vi "Aire (subVI).vi"(6 "milliseconds to wait":u32=2000, 8 "error in (no error)":errorcluster, 10 "Gas types":T1(array[ring])=[enum."TVOC", enum."H2S", enum."NO2", enum."O3", enum."SO2", enum."CO", enum."O2", enum."CO2"], 11 "Modbus Master in":refnum<class "Modbus Master.lvclass">) -> (0 "error out":errorcluster, 2 "Measures":dbl[](array[numeric]), 3 "Modbus Master out":refnum<class "Modbus Master.lvclass">)   [LabVIEW 2024]
uses:
  <vilib>/Modbus/master/Modbus Master.lvclass
  C:/Program Files (x86)/National Instruments/LabVIEW 2024/vi.lib/Modbus/subvis/Modbus API/Modbus API.lvclass
  <vilib>/Modbus/subvis/Modbus API/Modbus API.lvclass/Modbus API.ctl
  <vilib>/Modbus/subvis/Transmission Data Unit (ADU)/Transmission Data Unit/Transmission Data Unit.lvclass/Transmission Data Unit.ctl
  <vilib>/Modbus/master/Data Access/Unit ID/Set Unit ID Property.vi
  <vilib>/Modbus/subvis/Transmission Data Unit (ADU)/Transmission Data Unit/Data Access/Unit ID/Write Unit ID.vi
  <vilib>/Modbus/subvis/Modbus API/Read Transmission Data Unit.vi
  <vilib>/Modbus/subvis/Modbus API/Write Transmission Data Unit.vi
  <vilib>/Modbus/subvis/Transmission Data Unit (ADU)/Transmission Data Unit/Transmission Data Unit.lvclass
panel:
  out "element":u16
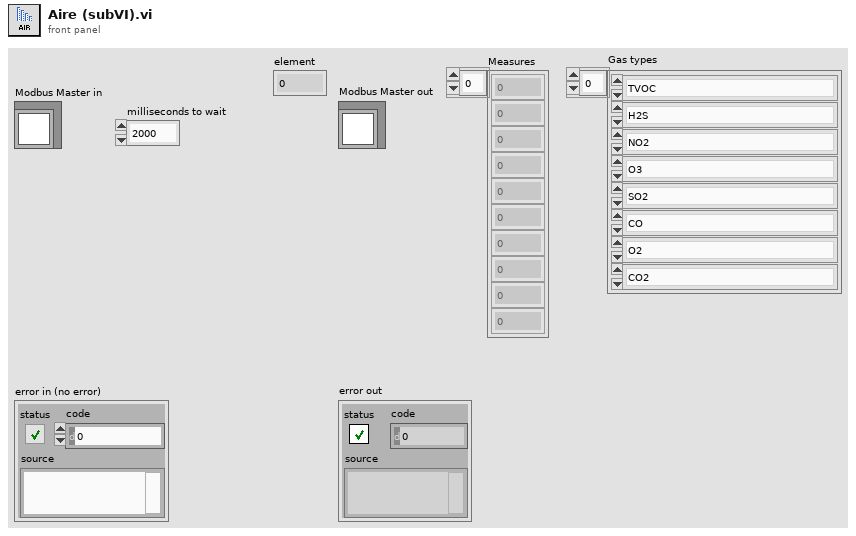
[diagram p1: front panel]
types:
  T1 = enum8{"TVOC", "H2S", "NO2", "O3", "SO2", "CO", "O2", "CO2"}[]
  T2 = enum8{"TVOC", "H2S", "NO2", "O3", "SO2", "CO", "O2", "CO2"}
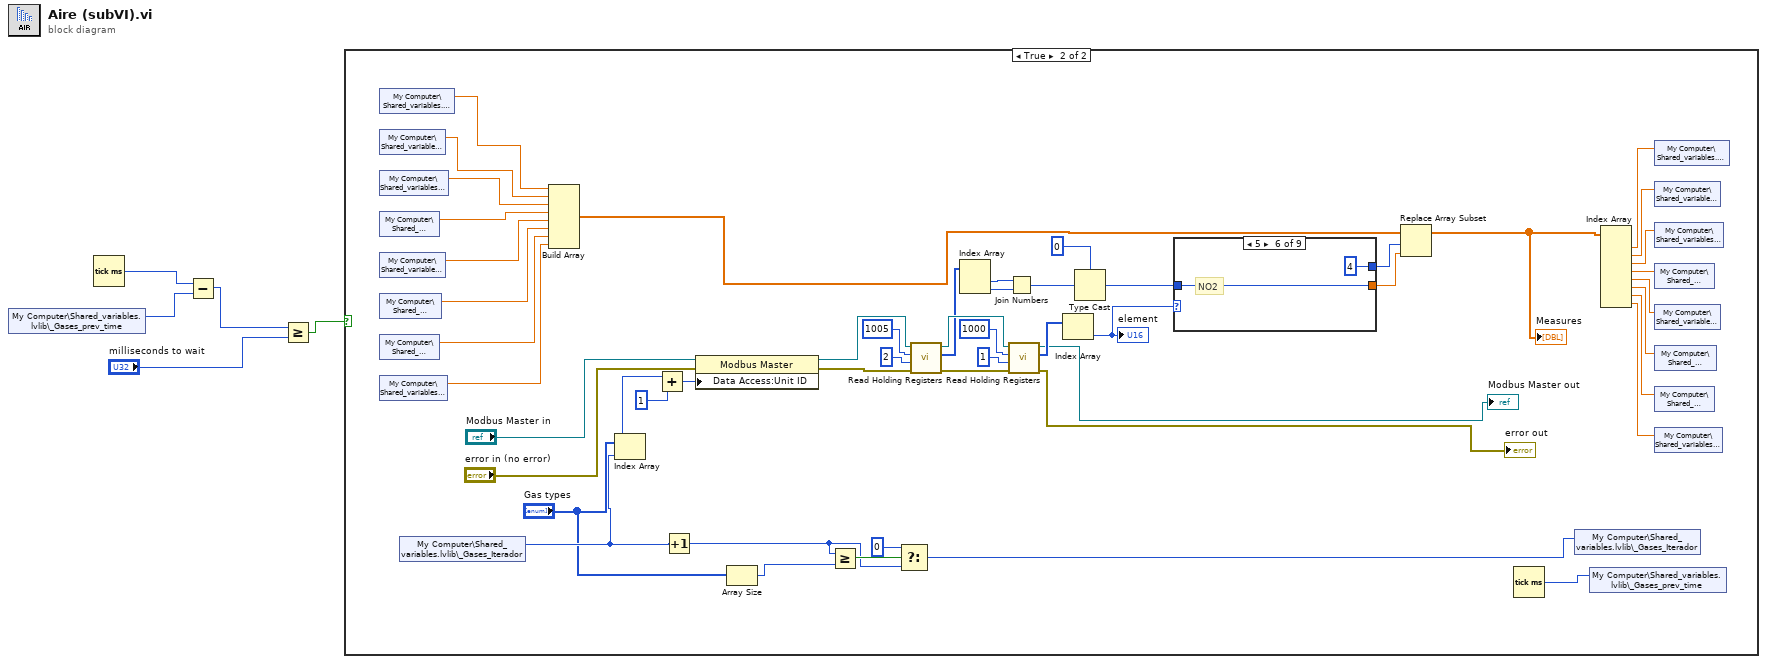
[diagram p0: block diagram]
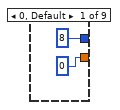
[diagram p3: hidden frame]
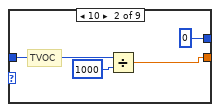
[diagram p4: hidden frame]
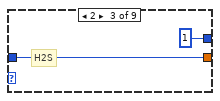
[diagram p5: hidden frame]
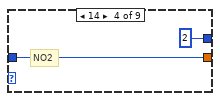
[diagram p6: hidden frame]
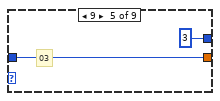
[diagram p7: hidden frame]
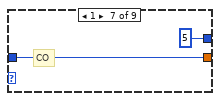
[diagram p8: hidden frame]
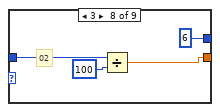
[diagram p9: hidden frame]
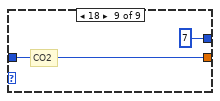
[diagram p10: hidden frame]
diagram:
  n1 = shared-variable "My Computer\\Shared_variables.lvlib\\_Gases_prev_time"() -> (w4:u32)  [unwired: 1 in, 1 out]
  n2 = Tick Count (ms)() -> (millisecond timer value=w5:u32)
  n3 = Subtract(x=w5, y=w4) -> (x-y=w3:u32)
  n4 = Greater Or Equal?(x=w3, y="milliseconds to wait") -> (x >= y?=w1:bool)
  n5 = case shown="True" w1 {
    frame False {
    }
    frame True {
      n6 = shared-variable "My Computer\\Shared_variables.lvlib\\TVOC"() -> (w48:dbl)  [unwired: 1 in, 1 out]
      n7 = shared-variable "My Computer\\Shared_variables.lvlib\\H2S"() -> (w47:dbl)  [unwired: 1 in, 1 out]
      n8 = shared-variable "My Computer\\Shared_variables.lvlib\\NO2"() -> (w46:dbl)  [unwired: 1 in, 1 out]
      n9 = shared-variable "My Computer\\Shared_variables.lvlib\\O3"() -> (w45:dbl)  [unwired: 1 in, 1 out]
      n10 = shared-variable "My Computer\\Shared_variables.lvlib\\SO2"() -> (w44:dbl)  [unwired: 1 in, 1 out]
      n11 = shared-variable "My Computer\\Shared_variables.lvlib\\CO"() -> (w43:dbl)  [unwired: 1 in, 1 out]
      n12 = shared-variable "My Computer\\Shared_variables.lvlib\\O2"() -> (w42:dbl)  [unwired: 1 in, 1 out]
      n13 = shared-variable "My Computer\\Shared_variables.lvlib\\CO2"() -> (w41:dbl)  [unwired: 1 in, 1 out]
      n14 = shared-variable "My Computer\\Shared_variables.lvlib\\_Gases_Iterador"() -> (w13:i8)  [unwired: 1 in, 1 out]
      n15 = Build Array(w48, w47, w46, w45, w44, w43, w42, w41) -> (w26:dbl[])
      n16 = Index Array(array="Gas types", index=w13) -> (element=w14:T2)
      n17 = Add(x=w14, y=1) -> (x+y=w27:u8)
      n18 = Increment(x=w13) -> (x+1=w8:i8)
      n19 = property class="Modbus Master"(reference="Modbus Master in", error in="error in (no error)", "Data Access:Unit ID"=w27) -> (reference out=w29:refnum<class "Modbus Master.lvclass">, error out=w30:errorcluster)
      n20 = Array Size(array="Gas types") -> (size(s)=w10:i32)
      n21 = Greater Or Equal?(x=w8, y=w10) -> (x >= y?=w9:bool)
      n22 = Select(t=i8 0, s=w9, f=w8) -> (s? t:f=w6:i8)
      n23 = call-dynamic "Read Holding Registers.vi"("error in (no error)"=w30, "number of holding registers"=u16 2, "starting address"=u16 1005, "Modbus master in"=w29) -> ("error out"=w35:errorcluster, "register values"=w31:u16[], "Modbus master out"=w34:refnum<class "Modbus Master.lvclass">)  [unwired: 5 in]
      n24 = Index Array(array=w31) -> (element #1=w32:u16, element #2=w33:u16)  [unwired: 2 in]
      n25 = Join Numbers(hi=w32, lo=w33) -> ((hi.lo)=w28:u32)
      n26 = call-dynamic "Read Holding Registers.vi"("error in (no error)"=w35, "number of holding registers"=u16 1, "starting address"=u16 1000, "Modbus master in"=w34) -> ("error out"=→"error out":errorcluster, "register values"=w36:u16[], "Modbus master out"=→"Modbus Master out":refnum<class "Modbus Master.lvclass">)  [unwired: 5 in]
      n27 = Index Array(array=w36) -> (element=w38:u16)  [unwired: 1 in]
      "element" <- w38
      n28 = Type Cast(type=0, x=w28) -> (*(type *) &x=w37:i32)
      n29 = case shown="5" w38 {
        tunnel: [8 ("index") 0 ("index") 1 ("index") 2 ("index") 3 ("index") 4 ("index") 5 ("index") 6 ("index") 7 ("index")] -> w40
        tunnel: [0 w60 w63 w65 w67 w69 w71 w73 w77] -> w39
        tunnel: w37 -> [_ w59 w63 w65 w67 w69 w71 w75 w77]
        frame 0, Default {
        }
        frame 10 {
          # "TVOC"
          n30 = Divide(x=w59, y=1000) -> (x/y=w60:dbl)
        }
        frame 2 {
          # "H2S"
        }
        frame 14 {
          # "NO2"
        }
        frame 9 {
          # "03"
        }
        frame 5 {
          # "NO2"
        }
        frame 1 {
          # "CO"
        }
        frame 3 {
          # "02"
          n31 = Divide(x=w75, y=100) -> (x/y=w73:dbl)
        }
        frame 18 {
          # "CO2"
        }
      }
      n32 = Replace Array Subset(array=w26, new element=w39, index=w40) -> (w17:dbl[])
      "Measures" <- w17
      n33 = Tick Count (ms)() -> (millisecond timer value=w12:u32)
      n34 = shared-variable "My Computer\\Shared_variables.lvlib\\_Gases_Iterador"(w6) -> ()  [unwired: 1 in, 1 out]
      n35 = shared-variable "My Computer\\Shared_variables.lvlib\\_Gases_prev_time"(w12) -> ()  [unwired: 1 in, 1 out]
      n36 = Index Array(array=w17) -> (element #1=w56:dbl, element #2=w55:dbl, element #3=w54:dbl, element #4=w53:dbl, element #5=w52:dbl, element #6=w51:dbl, element #7=w50:dbl, element #8=w49:dbl)  [unwired: 8 in]
      n37 = shared-variable "My Computer\\Shared_variables.lvlib\\TVOC"(w56) -> ()  [unwired: 1 in, 1 out]
      n38 = shared-variable "My Computer\\Shared_variables.lvlib\\H2S"(w55) -> ()  [unwired: 1 in, 1 out]
      n39 = shared-variable "My Computer\\Shared_variables.lvlib\\NO2"(w54) -> ()  [unwired: 1 in, 1 out]
      n40 = shared-variable "My Computer\\Shared_variables.lvlib\\O3"(w53) -> ()  [unwired: 1 in, 1 out]
      n41 = shared-variable "My Computer\\Shared_variables.lvlib\\SO2"(w52) -> ()  [unwired: 1 in, 1 out]
      n42 = shared-variable "My Computer\\Shared_variables.lvlib\\CO"(w51) -> ()  [unwired: 1 in, 1 out]
      n43 = shared-variable "My Computer\\Shared_variables.lvlib\\O2"(w50) -> ()  [unwired: 1 in, 1 out]
      n44 = shared-variable "My Computer\\Shared_variables.lvlib\\CO2"(w49) -> ()  [unwired: 1 in, 1 out]
    }
  }
